vi "Main_05b refactored.vi"() -> ()   [LabVIEW 2020]
panel:
  out "Answer":string
  out "Crate 2D Array":string[][](array[string])
  out "Starting Map (index 0 is top crate)":map{i32, string[]}(c390)
  out "Changing Map":map{i32, string[]}(c390)
  in  "Puzzle":string="[T] [V]                     [W]    \n[V] [C] [P] [D]             [B]    \n[J] [P] [R] [N] [B]         [Z]    \n[W] [Q] [D] [M] [T]     [L] [T]    \n[N] [J] [H] [B] [P] [T] [P] [L]    \n[R] [D] [F] [P] [R] [P] [R] [S] [G]\n[M] [W] [J] [R] [V] [B] [J] [C] [S]\n[S] [B] [B] [F] [H] [C] [B] [N] [L]\n 1   2   3   4   5   6   7   8   9 \n\nmove 7 from 3 to 9\nmove 6 from 2 to 1\nmove 2 from 4 to 8\nmove 10 from 8 to 4\nmove 1 from 2 to 4\nmove 15 from 4 to 1\nmove 28 from 1 to 3\nmove 1 from 2 to 5\nmove 7 from 5 to 9\nmove 5 from 9 to 5\nmove 21 from 3 to 1\nmove 1 from 6 to 4\nmove 4 from 9 to 2\nmove 7 from 9 to 2\nmove 4 from 2 to 6\nmove 1 from 9 to 1\nmove 2 from 4 to 9\nmove 2 from 7 to 4\nmove 4 from 3 to 5\nmove 2 from 7 to 9\nmove 5 from 2 to 7\nmove 2 from 9 to 1\nmove 1 from 9 to 2\nmove 3 from 3 to 7\nmove 3 from 5 to 2\nmove 2 from 6 to 1\nmove 1 from 9 to 4\nmove 25 from 1 to 9\nmove 2 from 5 to 3\nmove 1 from 1 to 7\nmove 9 from 7 to 1\nmove 1 from 2 to 8\nmove 16 from 9 to 7\nmove 5 from 9 to 5\nmove 7 from 1 to 8\nmove 1 from 9 to 7\nmove 18 from 7 to 4\nmove 1 from 3 to 4\nmove 1 from 1 to 8\nmove 2 from 8 to 1\nmove 1 from 3 to 9\nmove 17 from 4 to 5\nmove 5 from 8 to 6\nmove 2 from 8 to 1\nmove 6 from 6 to 7\nmove 2 from 9 to 4\nmove 5 from 1 to 3\nmove 3 from 3 to 7\nmove 1 from 1 to 2\nmove 2 from 3 to 8\nmove 2 from 4 to 1\nmove 2 from 8 to 7\nmove 2 from 9 to 7\nmove 1 from 2 to 4\nmove 1 from 2 to 4\nmove 2 from 1 to 7\nmove 11 from 7 to 1\nmove 4 from 4 to 1\nmove 3 from 1 to 3\nmove 7 from 1 to 8\nmove 4 from 2 to 8\nmove 2 from 1 to 4\nmove 2 from 4 to 3\nmove 2 from 1 to 3\nmove 3 from 7 to 4\nmove 4 from 8 to 6\nmove 1 from 7 to 5\nmove 2 from 4 to 1\nmove 4 from 6 to 2\nmove 3 from 1 to 8\nmove 6 from 8 to 6\nmove 1 from 2 to 1\nmove 23 from 5 to 8\nmove 21 from 8 to 3\nmove 2 from 6 to 9\nmove 1 from 8 to 9\nmove 2 from 3 to 7\nmove 26 from 3 to 8\nmove 2 from 9 to 2\nmove 8 from 6 to 3\nmove 3 from 5 to 4\nmove 1 from 7 to 4\nmove 1 from 7 to 9\nmove 1 from 5 to 4\nmove 5 from 2 to 9\nmove 7 from 9 to 8\nmove 38 from 8 to 7\nmove 1 from 1 to 7\nmove 1 from 4 to 9\nmove 3 from 4 to 1\nmove 4 from 3 to 2\nmove 1 from 1 to 7\nmove 34 from 7 to 6\nmove 3 from 4 to 7\nmove 1 from 4 to 2\nmove 2 from 1 to 3\nmove 1 from 2 to 9\nmove 5 from 3 to 6\nmove 1 from 4 to 6\nmove 4 from 2 to 6\nmove 1 from 9 to 5\nmove 4 from 7 to 3\nmove 1 from 5 to 9\nmove 1 from 9 to 1\nmove 1 from 3 to 6\nmove 1 from 9 to 3\nmove 5 from 7 to 9\nmove 1 from 1 to 9\nmove 3 from 9 to 1\nmove 1 from 3 to 4\nmove 38 from 6 to 1\nmove 2 from 9 to 4\nmove 3 from 3 to 6\nmove 1 from 9 to 5\nmove 8 from 6 to 8\nmove 1 from 3 to 6\nmove 1 from 6 to 8\nmove 2 from 4 to 3\nmove 4 from 8 to 5\nmove 1 from 6 to 2\nmove 1 from 2 to 7\nmove 1 from 6 to 3\nmove 3 from 8 to 7\nmove 4 from 7 to 6\nmove 1 from 4 to 1\nmove 5 from 1 to 4\nmove 4 from 6 to 5\nmove 3 from 5 to 8\nmove 3 from 5 to 3\nmove 1 from 8 to 2\nmove 6 from 3 to 8\nmove 1 from 5 to 7\nmove 1 from 2 to 1\nmove 1 from 7 to 6\nmove 3 from 4 to 9\nmove 6 from 8 to 6\nmove 3 from 8 to 2\nmove 3 from 6 to 2\nmove 1 from 4 to 5\nmove 1 from 6 to 9\nmove 2 from 6 to 1\nmove 1 from 4 to 1\nmove 2 from 5 to 2\nmove 1 from 8 to 5\nmove 1 from 9 to 8\nmove 22 from 1 to 5\nmove 3 from 2 to 3\nmove 1 from 8 to 4\nmove 2 from 3 to 6\nmove 1 from 6 to 4\nmove 1 from 3 to 8\nmove 1 from 2 to 8\nmove 10 from 5 to 3\nmove 1 from 6 to 8\nmove 2 from 8 to 4\nmove 1 from 6 to 3\nmove 2 from 2 to 3\nmove 1 from 8 to 5\nmove 13 from 3 to 4\nmove 2 from 1 to 7\nmove 11 from 1 to 2\nmove 3 from 4 to 5\nmove 6 from 1 to 9\nmove 8 from 2 to 6\nmove 4 from 2 to 1\nmove 2 from 6 to 5\nmove 4 from 1 to 8\nmove 2 from 8 to 6\nmove 1 from 7 to 1\nmove 1 from 7 to 2\nmove 8 from 6 to 5\nmove 1 from 8 to 4\nmove 1 from 1 to 6\nmove 10 from 5 to 1\nmove 3 from 9 to 4\nmove 6 from 1 to 3\nmove 9 from 4 to 5\nmove 1 from 2 to 1\nmove 1 from 4 to 9\nmove 1 from 6 to 8\nmove 1 from 2 to 1\nmove 1 from 4 to 8\nmove 2 from 8 to 9\nmove 1 from 8 to 6\nmove 1 from 3 to 2\nmove 1 from 1 to 4\nmove 1 from 2 to 5\nmove 1 from 1 to 8\nmove 1 from 6 to 8\nmove 8 from 5 to 3\nmove 1 from 8 to 7\nmove 1 from 7 to 8\nmove 6 from 9 to 6\nmove 2 from 9 to 2\nmove 1 from 9 to 7\nmove 1 from 8 to 5\nmove 1 from 2 to 7\nmove 1 from 2 to 9\nmove 16 from 5 to 2\nmove 4 from 5 to 1\nmove 12 from 3 to 6\nmove 1 from 5 to 4\nmove 8 from 6 to 9\nmove 1 from 8 to 5\nmove 2 from 9 to 6\nmove 2 from 2 to 5\nmove 3 from 1 to 4\nmove 3 from 6 to 7\nmove 7 from 9 to 6\nmove 4 from 7 to 1\nmove 1 from 5 to 2\nmove 1 from 3 to 2\nmove 4 from 1 to 9\nmove 4 from 9 to 5\nmove 12 from 6 to 7\nmove 4 from 2 to 6\nmove 4 from 2 to 9\nmove 7 from 6 to 3\nmove 3 from 9 to 8\nmove 5 from 2 to 4\nmove 4 from 5 to 7\nmove 1 from 9 to 4\nmove 13 from 7 to 8\nmove 3 from 7 to 8\nmove 2 from 3 to 2\nmove 5 from 1 to 5\nmove 11 from 4 to 9\nmove 7 from 9 to 1\nmove 4 from 4 to 3\nmove 1 from 6 to 8\nmove 8 from 8 to 4\nmove 1 from 1 to 7\nmove 3 from 4 to 6\nmove 4 from 2 to 8\nmove 3 from 5 to 4\nmove 1 from 4 to 1\nmove 4 from 9 to 8\nmove 3 from 5 to 2\nmove 2 from 2 to 3\nmove 1 from 6 to 7\nmove 7 from 1 to 9\nmove 3 from 7 to 4\nmove 1 from 4 to 2\nmove 1 from 6 to 8\nmove 1 from 5 to 7\nmove 1 from 6 to 7\nmove 9 from 4 to 6\nmove 7 from 9 to 5\nmove 1 from 4 to 3\nmove 1 from 5 to 6\nmove 4 from 3 to 7\nmove 3 from 3 to 1\nmove 2 from 2 to 4\nmove 3 from 1 to 6\nmove 4 from 5 to 1\nmove 2 from 5 to 3\nmove 3 from 6 to 8\nmove 6 from 7 to 3\nmove 10 from 3 to 7\nmove 10 from 6 to 4\nmove 3 from 1 to 9\nmove 4 from 7 to 2\nmove 2 from 3 to 5\nmove 1 from 3 to 5\nmove 1 from 1 to 2\nmove 3 from 9 to 1\nmove 2 from 1 to 9\nmove 4 from 2 to 5\nmove 10 from 4 to 9\nmove 2 from 8 to 7\nmove 1 from 2 to 9\nmove 1 from 9 to 4\nmove 1 from 1 to 9\nmove 3 from 7 to 8\nmove 5 from 9 to 8\nmove 6 from 5 to 4\nmove 5 from 9 to 6\nmove 5 from 8 to 5\nmove 4 from 5 to 2\nmove 3 from 7 to 8\nmove 3 from 9 to 1\nmove 2 from 5 to 8\nmove 1 from 4 to 6\nmove 3 from 6 to 3\nmove 8 from 4 to 3\nmove 2 from 6 to 7\nmove 24 from 8 to 9\nmove 1 from 6 to 9\nmove 8 from 9 to 3\nmove 1 from 1 to 9\nmove 2 from 8 to 3\nmove 3 from 9 to 4\nmove 18 from 3 to 5\nmove 1 from 2 to 6\nmove 1 from 6 to 1\nmove 13 from 9 to 8\nmove 3 from 4 to 1\nmove 1 from 4 to 2\nmove 1 from 5 to 3\nmove 1 from 9 to 2\nmove 6 from 2 to 9\nmove 3 from 3 to 1\nmove 3 from 7 to 6\nmove 2 from 1 to 5\nmove 3 from 6 to 7\nmove 17 from 8 to 1\nmove 8 from 5 to 7\nmove 11 from 7 to 5\nmove 1 from 4 to 5\nmove 24 from 1 to 3\nmove 7 from 5 to 9\nmove 11 from 5 to 9\nmove 1 from 5 to 4\nmove 1 from 5 to 2\nmove 1 from 4 to 7\nmove 16 from 3 to 1\nmove 3 from 5 to 8\nmove 1 from 9 to 1\nmove 12 from 9 to 2\nmove 5 from 3 to 1\nmove 2 from 8 to 5\nmove 2 from 3 to 4\nmove 1 from 8 to 6\nmove 2 from 5 to 3\nmove 1 from 6 to 1\nmove 2 from 4 to 1\nmove 8 from 2 to 1\nmove 24 from 1 to 6\nmove 1 from 9 to 6\nmove 4 from 2 to 6\nmove 4 from 3 to 2\nmove 4 from 9 to 4\nmove 1 from 7 to 5\nmove 6 from 9 to 1\nmove 17 from 6 to 4\nmove 1 from 1 to 9\nmove 2 from 9 to 7\nmove 9 from 6 to 7\nmove 12 from 7 to 2\nmove 11 from 1 to 2\nmove 12 from 4 to 2\nmove 1 from 1 to 4\nmove 1 from 5 to 7\nmove 2 from 6 to 3\nmove 2 from 4 to 3\nmove 1 from 1 to 6\nmove 5 from 4 to 2\nmove 1 from 7 to 5\nmove 2 from 6 to 9\nmove 6 from 2 to 4\nmove 1 from 5 to 8\nmove 3 from 4 to 1\nmove 1 from 8 to 9\nmove 5 from 4 to 1\nmove 1 from 1 to 2\nmove 1 from 3 to 8\nmove 7 from 1 to 6\nmove 1 from 8 to 6\nmove 1 from 3 to 5\nmove 1 from 1 to 8\nmove 1 from 4 to 5\nmove 2 from 5 to 9\nmove 1 from 8 to 2\nmove 2 from 6 to 8\nmove 1 from 8 to 6\nmove 1 from 6 to 8\nmove 1 from 8 to 5\nmove 4 from 9 to 5\nmove 1 from 9 to 6\nmove 1 from 6 to 8\nmove 37 from 2 to 5\nmove 1 from 2 to 8\nmove 37 from 5 to 8\nmove 21 from 8 to 4\nmove 1 from 3 to 7\nmove 12 from 4 to 1\nmove 1 from 7 to 8\nmove 4 from 6 to 3\nmove 1 from 4 to 2\nmove 2 from 2 to 6\nmove 2 from 3 to 2\nmove 2 from 2 to 7\nmove 2 from 7 to 1\nmove 3 from 5 to 3\nmove 2 from 2 to 8\nmove 15 from 8 to 7\nmove 1 from 7 to 2\nmove 2 from 5 to 8\nmove 5 from 4 to 3\nmove 3 from 6 to 2\nmove 8 from 1 to 9\nmove 8 from 9 to 4\nmove 7 from 8 to 9\nmove 2 from 8 to 5\nmove 4 from 1 to 9\nmove 10 from 3 to 2\nmove 1 from 6 to 7\nmove 6 from 7 to 8\nmove 10 from 4 to 7\nmove 1 from 3 to 7\nmove 3 from 9 to 1\nmove 5 from 8 to 1\nmove 5 from 2 to 7\nmove 1 from 4 to 3\nmove 1 from 5 to 6\nmove 10 from 1 to 7\nmove 34 from 7 to 4\nmove 1 from 6 to 9\nmove 1 from 7 to 3\nmove 8 from 4 to 2\nmove 1 from 9 to 7\nmove 1 from 7 to 9\nmove 22 from 4 to 5\nmove 1 from 3 to 8\nmove 6 from 5 to 6\nmove 1 from 8 to 4\nmove 9 from 9 to 4\nmove 1 from 3 to 2\nmove 4 from 2 to 1\nmove 11 from 2 to 6\nmove 14 from 4 to 7\nmove 1 from 2 to 1\nmove 12 from 5 to 6\nmove 7 from 7 to 9\nmove 2 from 5 to 4\nmove 1 from 8 to 5\nmove 6 from 6 to 8\nmove 3 from 7 to 8\nmove 1 from 2 to 6\nmove 2 from 4 to 3\nmove 1 from 3 to 8\nmove 1 from 2 to 5\nmove 1 from 3 to 4\nmove 5 from 8 to 9\nmove 5 from 1 to 4\nmove 3 from 8 to 9\nmove 5 from 4 to 7\nmove 18 from 6 to 3\nmove 2 from 8 to 9\nmove 3 from 6 to 3\nmove 5 from 7 to 1\nmove 1 from 6 to 7\nmove 3 from 9 to 7\nmove 6 from 7 to 8\nmove 8 from 9 to 8\nmove 1 from 7 to 6\nmove 12 from 3 to 1\nmove 2 from 9 to 7\nmove 1 from 8 to 6\nmove 9 from 8 to 9\nmove 2 from 8 to 7\nmove 1 from 7 to 8\nmove 2 from 1 to 6\nmove 7 from 1 to 9\nmove 16 from 9 to 5\nmove 4 from 3 to 9\nmove 8 from 1 to 3\nmove 5 from 5 to 1\nmove 1 from 4 to 3\nmove 4 from 7 to 6\nmove 3 from 8 to 2\nmove 8 from 3 to 2\nmove 11 from 2 to 7\nmove 3 from 6 to 1\nmove 4 from 3 to 6\nmove 12 from 5 to 7\nmove 2 from 3 to 6\nmove 7 from 1 to 7\nmove 2 from 5 to 1\nmove 1 from 9 to 2\nmove 1 from 5 to 7\nmove 31 from 7 to 4\nmove 6 from 9 to 1\nmove 6 from 4 to 7\nmove 16 from 4 to 5\nmove 1 from 9 to 4\nmove 1 from 7 to 6\nmove 4 from 4 to 1\nmove 11 from 5 to 9\nmove 2 from 5 to 6\nmove 1 from 2 to 9\nmove 4 from 5 to 1\nmove 8 from 9 to 2\nmove 12 from 6 to 5\nmove 11 from 5 to 1\nmove 18 from 1 to 2\nmove 3 from 4 to 3\nmove 2 from 6 to 7\nmove 2 from 9 to 1\nmove 1 from 5 to 9\nmove 3 from 9 to 5\nmove 13 from 2 to 8\nmove 10 from 8 to 2\nmove 3 from 8 to 6\nmove 3 from 3 to 9\nmove 7 from 1 to 5\nmove 6 from 5 to 6\nmove 3 from 1 to 2\nmove 5 from 7 to 8\nmove 13 from 2 to 8\nmove 9 from 6 to 3"
  in  "Example":string=" [D]    \n[N] [C]    \n[Z] [M] [P]\n 1   2   3 \n\nmove 1 from 2 to 1\nmove 3 from 1 to 3\nmove 2 from 2 to 1\nmove 1 from 1 to 2"
  # "--- Part Two ---\nAs you watch the crane operator expertly rearrange the crates, you notice the process isn't following your prediction.\n\nSome mud was covering the writing on the side of the crane, and you quickly wipe it away. The crane isn't a CrateMover 9000 - it's a CrateMover 9001.\n\nThe CrateMover 9001 is notable for many new and exciting features: air conditioning, leather seats, an extra cup holder, and the ability to pick up and move multiple crates at once.\n\nAgain considering the example above, the crates begin in the same configuration:\n\n    [D]    \n[N] [C]    \n[Z] [M] [P]\n 1   2   3 \nMoving a single crate from stack 2 to stack 1 behaves the same as before:\n\n[D]        \n[N] [C]    \n[Z] [M] [P]\n 1   2   3 \nHowever, the action of moving three crates from stack 1 to stack 3 means that those three moved crates stay in the same order, resulting in this new configuration:\n\n        [D]\n        [N]\n    [C] [Z]\n    [M] [P]\n 1   2   3\nNext, as both crates are moved from stack 2 to stack 1, they retain their order as well:\n\n        [D]\n        [N]\n[C]     [Z]\n[M]     [P]\n 1   2   3\nFinally, a single crate is still moved from stack 1 to stack 2, but now it's crate C that gets moved:\n\n        [D]\n        [N]\n        [Z]\n[M] [C] [P]\n 1   2   3\nIn this example, the CrateMover 9001 has put the crates in a totally different order: MCD.\n\nBefore the rearrangement process finishes, update your simulation so that the Elves know where they should stand to be ready to unload the final supplies. After the rearrangement procedure completes, what crate ends up on top of each stack?"
  # "BRQWDBBJM"
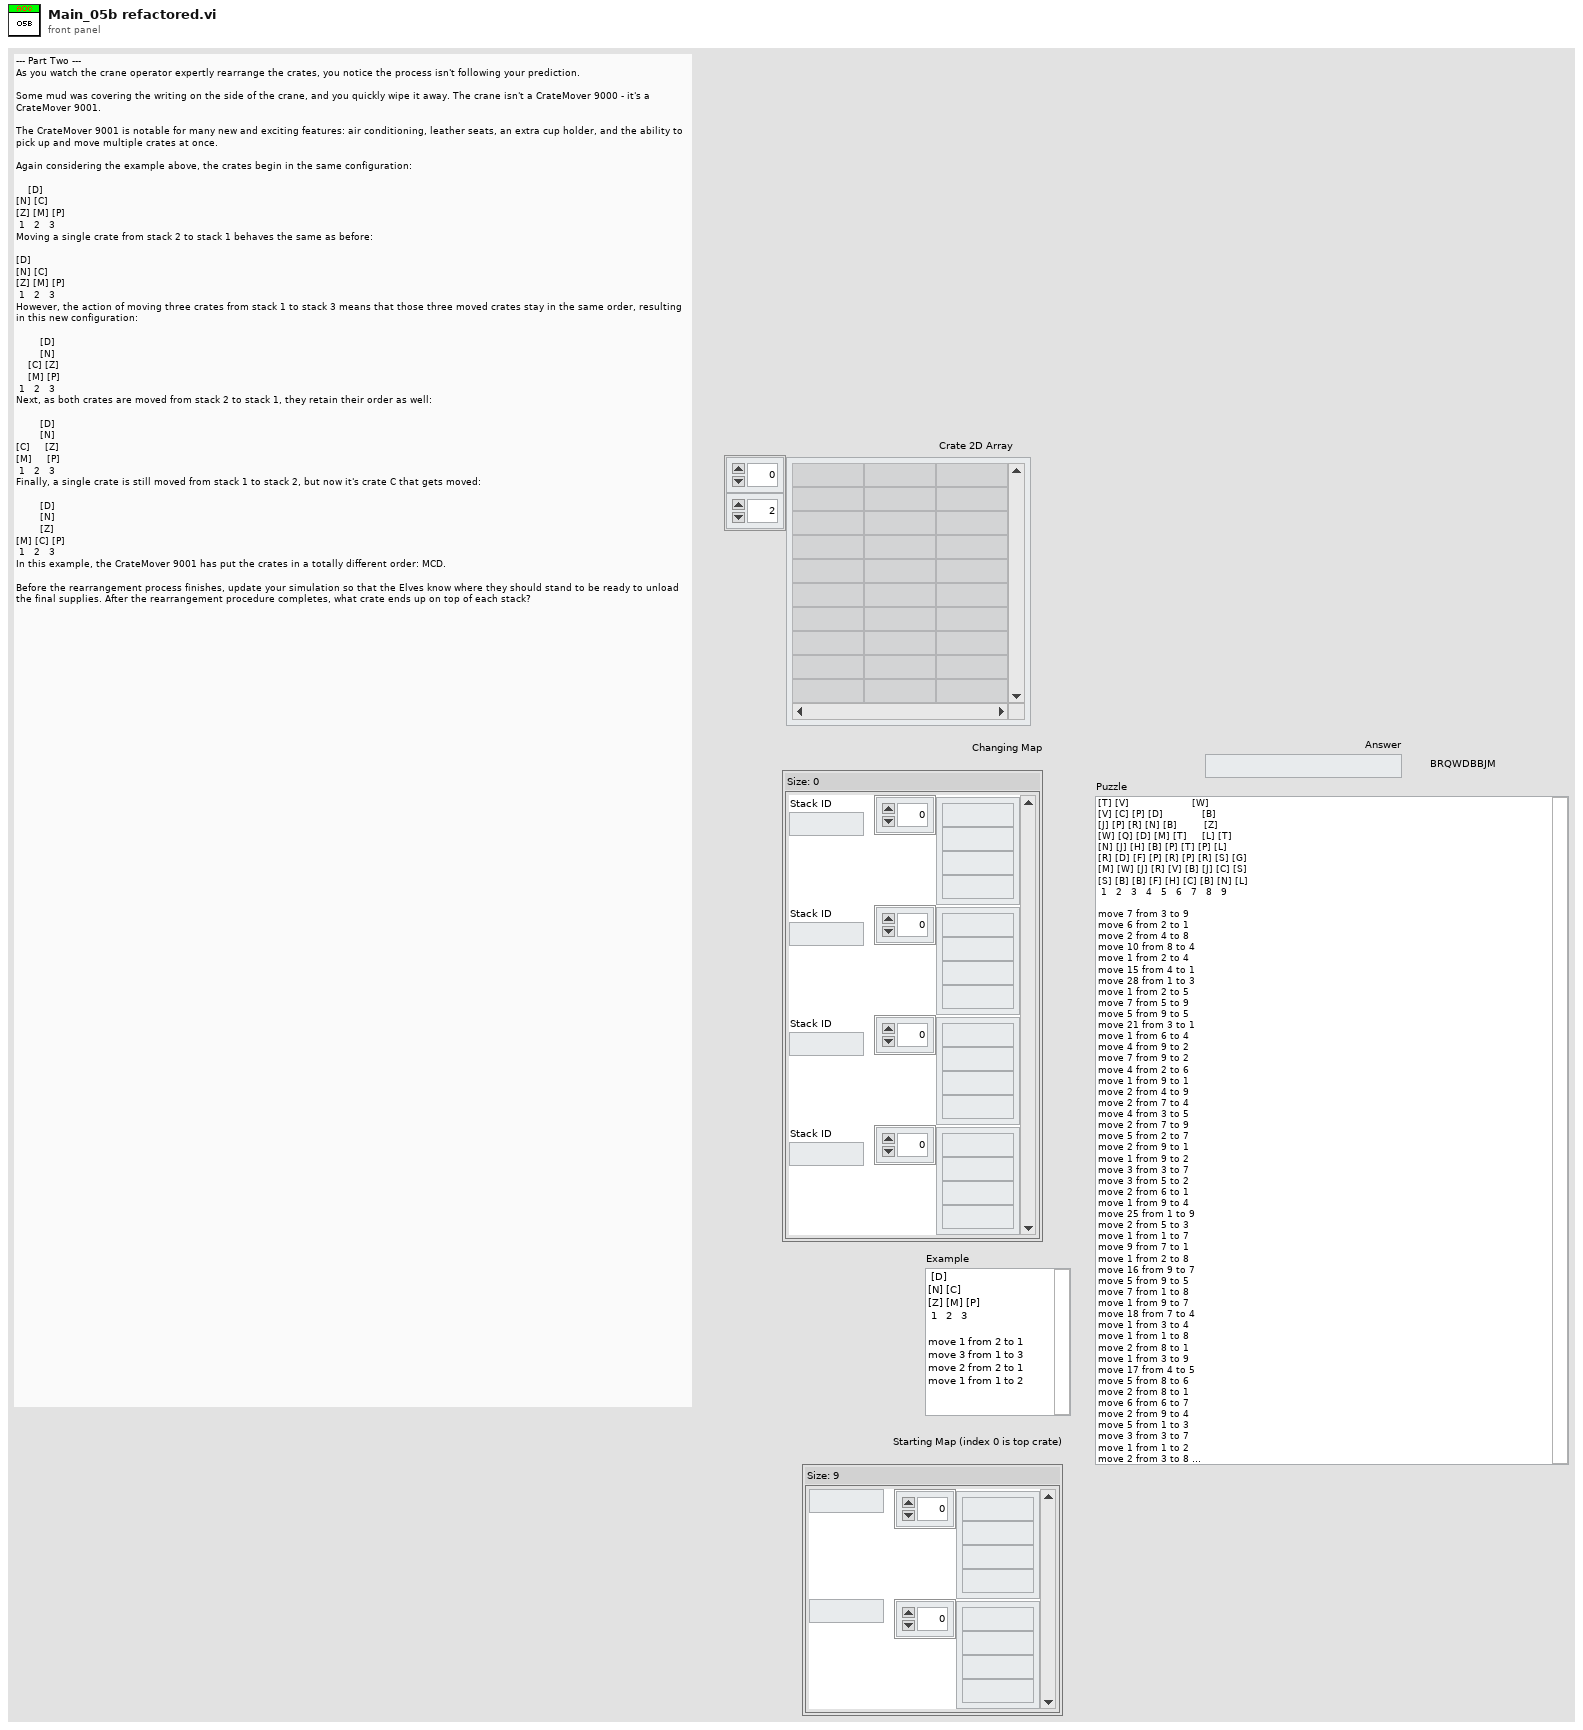
[diagram p1: front panel]
types:
  T1 = cluster{"Count":i32, "Start Pile":i32, "End Pile":i32}
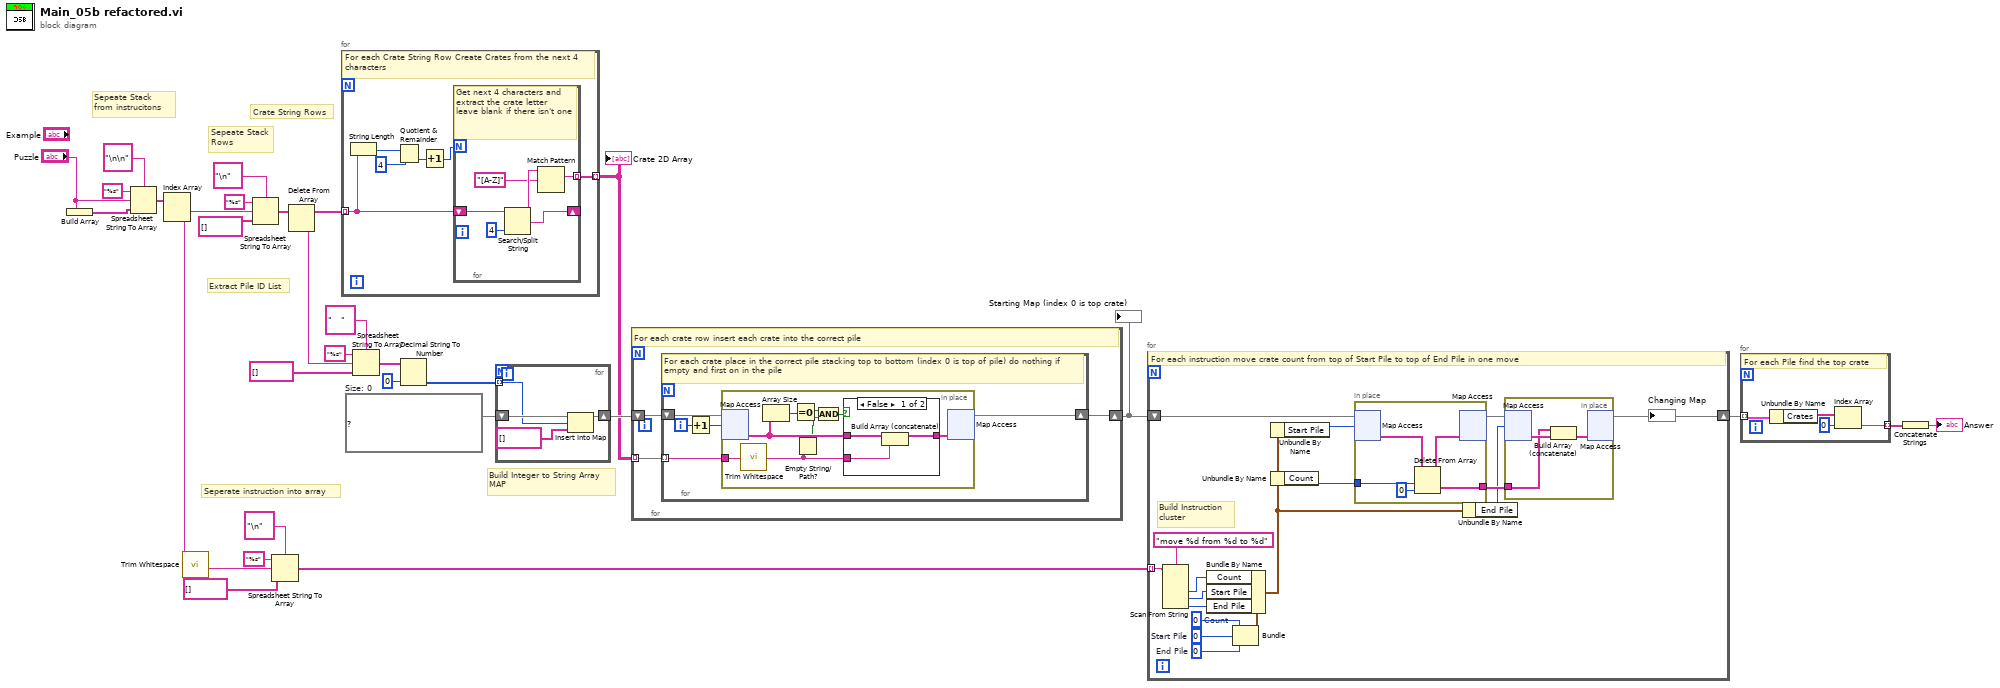
[diagram p0: block diagram]
diagram:
  w18 = map{i32, string[]} {}  # Size: 0
  # "Seperate instruction into array"
  # "Build Integer to String Array\nMAP"
  # "Crate String Rows"
  # "Extract Pile ID List"
  # "Sepeate Stack\nRows"
  # "Sepeate Stack\nfrom instrucitons"
  n1 = Build Array("Puzzle") -> (w31:string[])
  n2 = Spreadsheet String To Array(delimiter (Tab)="\n\n", format string="%s", spreadsheet string="Puzzle", array type (2D Dbl)=w31) -> (array=w28:string[])
  n3 = Index Array(array=w28) -> (element #1=w25:string, element #2=w15:string)  [unwired: 2 in]
  n4 = call <vilib>:"Trim Whitespace.vi"("string"=w15) -> ("trimmed string"=w12:string)  [unwired: 1 in]
  n5 = Spreadsheet String To Array(delimiter (Tab)="\n", format string="%s", spreadsheet string=w25, array type (2D Dbl)=string[] [] ("appended array")) -> (array=w24:string[])
  n6 = Spreadsheet String To Array(delimiter (Tab)="\n", format string="%s", spreadsheet string=w12, array type (2D Dbl)=string[] [] ("value")) -> (array=w10:string[])
  n7 = Delete From Array(array=w24) -> (deleted portion=w21:string, array with subset deleted=w8:string[])  [unwired: 2 in]
  n8 = for {
    tunnel: w8 -> [w34] mode=indexing
    tunnel: [w33] -> w7 mode=indexing
    # "For each Crate String Row Create Crates from the next 4 characters"
    n9 = String Length(string=w34) -> (length=w37:i32)
    n10 = Quotient & Remainder(x=w37, y=4) -> (floor(x/y)=w35:i32)  [unwired: 1 out]
    n11 = Increment(x=w35) -> (x+1=w32:i32)
    n12 = for {
      N: w32 -> [_]
      shift-right: [w42] -> _
      shift-left: w34 -> [w43]
      tunnel: [w38] -> w33 mode=indexing
      # "Get next 4 characters and extract the crate letter leave blank if there isn't one"
      n13 = Search/Split String(string=w43, offset (0)=4) -> (substring before match=w40:string, match + rest of string=w42:string)  [unwired: 1 in, 1 out]
      n14 = Match Pattern(string=w40, regular expression="[A-Z]") -> (match substring=w38:string)  [unwired: 1 in, 3 out]
    }
  }
  "Crate 2D Array" <- w7
  n15 = Spreadsheet String To Array(delimiter (Tab)="   ", format string="%s", spreadsheet string=w21, array type (2D Dbl)=string[] [] ("appended array")) -> (array=w20:string[])
  n16 = Decimal String To Number(string=w20, default (0L)=0 ("default (0 I32)")) -> (number=w17:i32[])  [unwired: 1 in, 1 out]
  n17 = for {
    shift-right: [w46] -> w16
    shift-left: w18 -> [w47]
    tunnel: w17 -> [w44] mode=indexing
    n18 = Insert Into Map(map in=w47, key=w44, value=string[] []) -> (map out=w46:map{i32, string[]})  [unwired: 2 out]
  }
  n19 = for {
    shift-right: [w48] -> w9
    shift-left: w16 -> [w50]
    tunnel: w7 -> [w49] mode=indexing
    # "For each crate row insert each crate into the correct pile"
    n20 = for {
      shift-right: [w52] -> w48
      shift-left: w50 -> [w55]
      tunnel: w49 -> [w51] mode=indexing
      i -> [w54]
      # "For each crate place in the correct pile stacking top to bottom (index 0 is top of pile) do nothing if empty and first on in the pile"
      n21 = Increment(x=w54) -> (x+1=w53:i32)
      n22 = in-place {
        in-place-border: w51 -> [w60]
        n23 = in-place-map #1(w55, w53) -> (w62:string[])  [unwired: 1 in, 1 out]
        n24 = call <vilib>:"Trim Whitespace.vi"("string"=w60) -> ("trimmed string"=w59:string)  [unwired: 1 in]
        n25 = Array Size(array=w62) -> (size(s)=w61:i32)
        n26 = Equal To 0?(x=w61) -> (x = 0?=w57:bool)
        n27 = Empty String/Path?(string/path=w59) -> (empty?=w58:bool)
        n28 = And(x=w57, y=w58) -> (x .and. y?=w56:bool)
        n29 = case shown="False" w56 {
          tunnel: [w66 w67] -> w63
          tunnel: w59 -> [w65 _]
          tunnel: w62 -> [w64 w67]
          frame False {
            n30 = Build Array (concatenate)(w64, w65) -> (w66:string[])
          }
          frame True {
          }
        }
        n31 = in-place-map #1(w63) -> (w52:map{i32, string[]})  [unwired: 1 in, 2 out]
      }
    }
  }
  "Starting Map (index 0 is top crate)" <- w9
  n32 = for {
    tunnel: w10 -> [w76] mode=indexing
    shift-right: [w72] -> w6
    shift-left: w9 -> [w75]
    w84 = 0  # End Pile
    w80 = 0  # Count
    w83 = 0  # Start Pile
    # "Build Instruction\ncluster"
    # "For each instruction move crate count from top of Start Pile to top of End Pile in one move"
    n33 = Scan From String(format string="move %d from %d to %d", input string=w76) -> (output 1=w78:i32, output 2=w79:i32, output 3=w77:i32)  [unwired: 5 in, 3 out]
    n34 = Bundle("Count"=w80, "Start Pile"=w83, "End Pile"=w84) -> (w81:T1)  [unwired: 1 in]
    n35 = Bundle By Name(cluster=w81, "Count"=w78, "Start Pile"=w79, "End Pile"=w77) -> (w73:T1)
    n36 = Unbundle By Name(w73) -> ("Start Pile"=w74:i32)
    n37 = Unbundle By Name(w73) -> ("Count"=w68:i32)
    n38 = in-place {
      in-place-border: [w89] -> w70
      in-place-border: w68 -> [w88]
      n39 = in-place-map #2(w75, w74) -> (w92:string[])  [unwired: 1 in, 1 out]
      n40 = Delete From Array(array=w92, length=w88, index=0) -> (deleted portion=w89:string[], array with subset deleted=w91:string[])
      n41 = in-place-map #2(w91) -> (w71:map{i32, string[]})  [unwired: 1 in, 2 out]
    }
    n42 = Unbundle By Name(w73) -> ("End Pile"=w69:i32)
    n43 = in-place {
      in-place-border: w70 -> [w85]
      n44 = in-place-map #3(w71, w69) -> (w87:string[])  [unwired: 1 in, 1 out]
      n45 = Build Array (concatenate)(w85, w87) -> (w86:string[])
      n46 = in-place-map #3(w86) -> (w72:map{i32, string[]})  [unwired: 1 in, 2 out]
    }
    "Changing Map" <- w72
  }
  n47 = for {
    tunnel: w6 -> [w96] mode=indexing
    tunnel: [w94] -> w5 mode=indexing
    # "For each Pile find the top crate"
    n48 = Unbundle By Name(w96) -> ("Crates"=w95:string[])
    n49 = Index Array(array=w95, index=0) -> (element=w94:string)
  }
  n50 = Concatenate Strings(w5) -> (→"Answer":string)
